vi "Init.vi"(4 "Debug (F)":bool, 7 "Options (None)":T2, 8 "error in (no error)":errorcluster, 10 "Dynamic Values":refnum<class "Dynamic Values.lvclass">, 11 "Combobox":refnum<vi>) -> (0 "error out":errorcluster, 3 "Dynamic Combobox out":refnum<class "Dynamic Combobox.lvclass">, 5 "Dynamic Combobox Events":T1)   [LabVIEW 2020, in "Dynamic Combobox.lvlib" / "Dynamic Combobox.lvclass"]
doc: "Initializes a new instance of the Dynamic Combobox API for a specified <b>Combobox</b> and <b>Dynamic Values</b> instance. <b>Dynamic Values</b> is any class that inherits from the Dynamic Values interface to be able to provide the list of Strings and Values to display in the <b>Combobox</b>\n\n<b>Debug</b> can be set to True to have the Event Loop.vi front panel displayed when it runs so that it can be debugged if there are issues.\n\n<b>Browse Entry</b> adds an element to the selection menu for the combobox to use a search/list UI to select a value. This can be handy for long selection lists. It's also possible for different Dynamic Values implementations to provide their own specific browse UI.\n\n<b>Refresh Entry</b> adds an element to the selection menu to allow the user to update the selection list."
uses:
  Dynamic Combobox.lvclass
  Dynamic Values/Dynamic Values.lvclass
  Options.ctl
  Dynamic Combobox Events.ctl
  Ref Data.ctl
  <vilib>/Utility/miscctls.llb/LVComboBoxStrsAndValuesArrayTypeDef.ctl
  Dynamic Combobox.lvclass/Dynamic Combobox.ctl
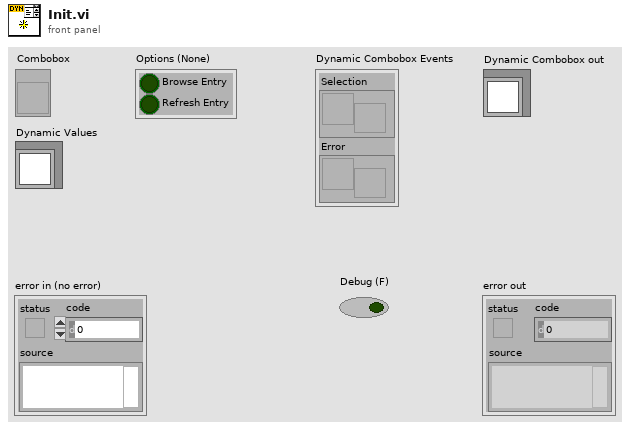
[diagram p1: front panel]
types:
  T1 = typedef "Dynamic Combobox.lvlib/Dynamic Combobox.lvclass/Dynamic Combobox Events.ctl" = cluster{"Selection":refnum<user-event>, "Error":refnum<user-event>}
  T2 = typedef "Dynamic Combobox.lvlib/Dynamic Combobox.lvclass/Options.ctl" = cluster{"Browse Entry":bool, "Refresh Entry":bool}
  T3 = typedef "Dynamic Combobox.lvlib/Dynamic Combobox.lvclass/Ref Data.ctl" = cluster{"Values":refnum<class "Dynamic Values.lvclass">, "Debug":bool, "Strings And Values []":T4, "Options":T2}
  T4 = typedef "LVComboBoxStrsAndValuesArrayTypeDef.ctl" = cluster{"String":string, "Value":string}[]
  T5 = enum8{"Enabled", "Disabled", "Disabled and Grayed Out"}
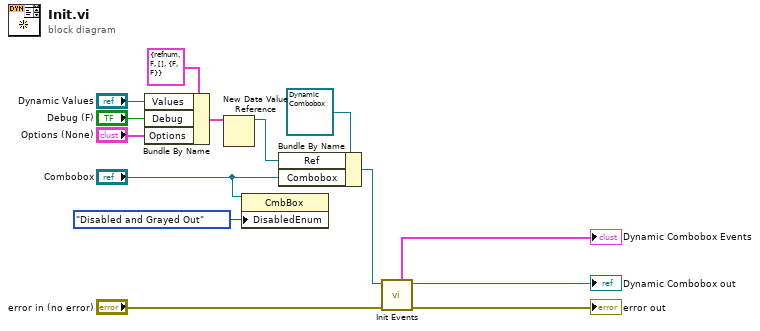
[diagram p0: block diagram]
diagram:
  n1 = Bundle By Name(cluster=T3 {"Values"=refnum, "Debug"=FALSE, "Strings And Values []"=[], "Options"={"Browse Entry"=FALSE, "Refresh Entry"=FALSE}} ("Ref Data"), "Values"="Dynamic Values", "Debug"="Debug (F)", "Options"="Options (None)") -> (w5:T3)
  n2 = New Data Value Reference(data value=w5) -> (data value reference=w4:refnum<data-value>)  [unwired: 1 in, 1 out]
  n3 = property class="CmbBox"(reference="Combobox", "DisabledEnum"=T5."Disabled and Grayed Out" ("Disabled")) -> ()  [unwired: 1 in, 2 out]
  n4 = Bundle By Name(cluster=refnum<class "Dynamic Combobox.lvclass"> refnum ("Dynamic Combobox in"), "Ref"=w4, "Combobox"="Combobox") -> (w12:refnum<class "Dynamic Combobox.lvclass">)
  n5 = call "Init Events.vi"("error in (no error)"="error in (no error)", "Dynamic Combobox in"=w12) -> ("error out"=→"error out":errorcluster, "Dynamic Combobox out"=→"Dynamic Combobox out":refnum<class "Dynamic Combobox.lvclass">, "External Events"=→"Dynamic Combobox Events":T1)  [unwired: 7 in]
